vi "U64_Read Index.vi"(9 "Default":u64, 11 "Index":i32) -> (1 "Value":u64)   [LabVIEW 2010, in "Current Value Table.lvlib"]
doc: "This VI takes a memory index (I32) and will perform a read on that index. This VI will never return the default value, as it has no error handling for increased performance. If the index is invalid, the default for the data type will be returned."
uses:
  Current Value Table.lvlib
  Type Defs/Memory Commands.ctl
  U64_Memory Block.vi
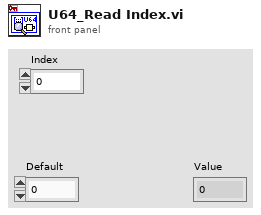
[diagram p1: front panel]
types:
  T1 = typedef "Current Value Table.lvlib/Memory Commands.ctl" = enum16{"Init", "Add Data", "Read", "Read Group", "Read All", "Write", "Write Group", "Get Size"}
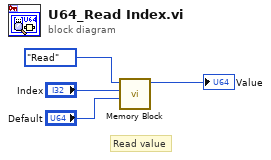
[diagram p0: block diagram]
diagram:
  # "Read value"
  n1 = call-poly "Memory Block.vi"("Value"="Default", "Index"="Index", "Method"=Memory_Commands."Read") -> ("Value Out"=→"Value":u64)  [unwired: 6 in, 2 out]
